vi "execute.vi"(8 "error in (no error)":errorcluster, 9 "daq in":refnum<class "GenericComponent.lvclass">, 10 "imaging mode in":refnum<class "GenericComponent.lvclass">, 11 "AdapterDL091215ImagingModeToDAQ in":refnum<class "AdapterDL091215ImagingModeToDAQ.lvclass">) -> (0 "error out":errorcluster, 1 "daq out":refnum<class "GenericComponent.lvclass">, 2 "imaging mode out":refnum<class "GenericComponent.lvclass">, 3 "AdapterDL091215ImagingModeToDAQ out":refnum<class "AdapterDL091215ImagingModeToDAQ.lvclass">)   [LabVIEW 2010, in "AdapterDL091215ImagingModeToDAQ.lvclass"]
uses:
  AdapterDL091215ImagingModeToDAQ.lvclass
  common/classes/GenericComponent/GenericComponent/GenericComponent.lvclass
  DAQ/DAQ_MG090622Camera/DAQ_MG090622Camera/DAQ_MG090622Camera.lvclass
  ImagingMode/ImagingModeMG091111IntrinsicImaging/ImagingModeMG091111IntrinsicImaging/ImagingModeMG091111IntrinsicImaging.lvclass
panel:
  # "imaging mode: ImagingModeMG091111IntrinsicImaging\nDAQ: DAQ_MG090622Camera"
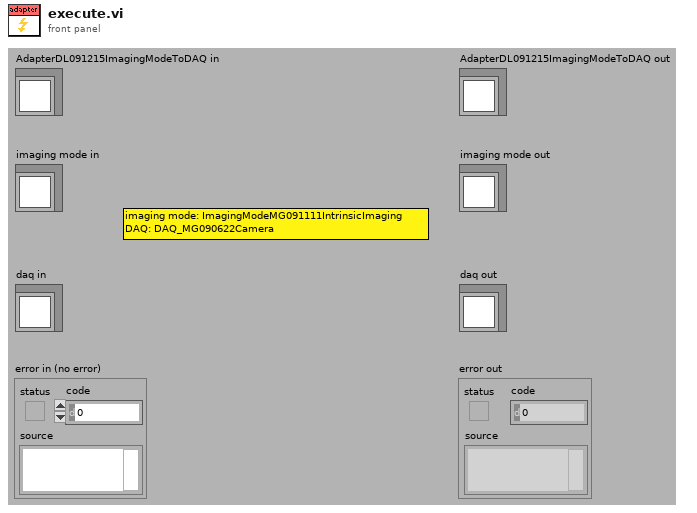
[diagram p1: front panel]
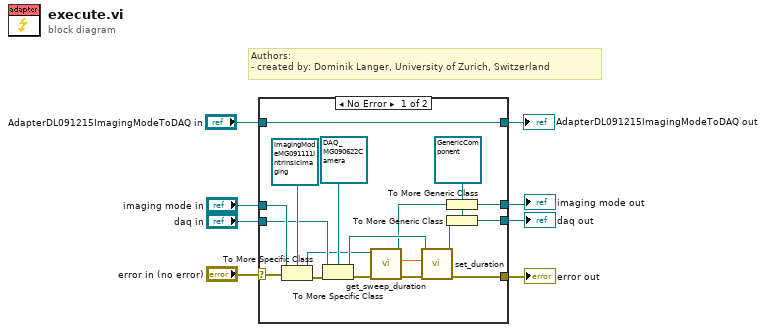
[diagram p0: block diagram]
diagram:
  # "Authors: \n- created by: Dominik Langer, University of Zurich, Switzerland"
  n1 = case shown="No Error" "error in (no error)" {
    selector: "error in (no error)" -> [w26 w28]
    tunnel: "imaging mode in" -> [w25 w29]
    tunnel: "AdapterDL091215ImagingModeToDAQ in" -> [w24 w30]
    tunnel: [w24 w30] -> w5
    tunnel: "daq in" -> [w21 w27]
    tunnel: [w19 w29] -> w3
    tunnel: [w17 w27] -> w2
    tunnel: [w15 w28] -> w1
    frame No Error {
      w18 = refnum<class "GenericComponent.lvclass"> refnum ("GenericComponent.lvclass")
      n2 = To More Specific Class(target class=refnum<class "ImagingModeMG091111IntrinsicImaging.lvclass"> refnum ("ImagingModeMG091111IntrinsicImaging.lvclass"), reference=w25, error in=w26) -> (specific class reference=w12:refnum<class "ImagingModeMG091111IntrinsicImaging.lvclass">, error out=w22:errorcluster)
      n3 = To More Specific Class(target class=refnum<class "DAQ_MG090622Camera.lvclass"> refnum ("DAQ_MG090622Camera.lvclass"), reference=w21, error in=w22) -> (specific class reference=w16:refnum<class "DAQ_MG090622Camera.lvclass">, error out=w13:errorcluster)
      n4 = call-dynamic "get_sweep_duration.vi"("error in (no error)"=w13, "ScanModeMG091111IntrinsicImaging in"=w12) -> ("error out"=w11:errorcluster, "sweep duration"=w10:dbl[unit], "ScanModeMG091111IntrinsicImaging out"=w9:refnum<class "ImagingModeMG091111IntrinsicImaging.lvclass">)  [unwired: 7 in]
      n5 = call-dynamic "set_duration.vi"("error in (no error)"=w11, "duration"=w10, "DAQ_MG090622Camera in"=w16) -> ("error out"=w15:errorcluster, "DAQ_MG090622Camera out"=w14:refnum<class "DAQ_MG090622Camera.lvclass">)  [unwired: 7 in]
      n6 = To More Generic Class(target class=w18, reference=w9) -> (generic class reference=w19:refnum<class "GenericComponent.lvclass">)
      n7 = To More Generic Class(target class=w18, reference=w14) -> (generic class reference=w17:refnum<class "GenericComponent.lvclass">)
    }
    frame Error {
    }
  }
  "error out" <- w1
  "AdapterDL091215ImagingModeToDAQ out" <- w5
  "imaging mode out" <- w3
  "daq out" <- w2
